vi "Create Event List.vi"(10 "Event Outcome":T1, 11 "Array in":T1[](array[typedef])) -> (3 "Array out":T1[](array[typedef]))   [LabVIEW 2017]
uses:
  state-manager/Event.ctl
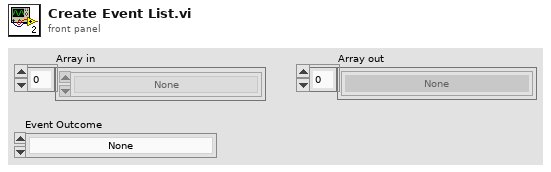
[diagram p1: front panel]
types:
  T1 = typedef "Event.ctl" = enum16{"None", "Zig Zag Finished", "Start Obstacle Avoidance", "Start Button Pressed", "Black & Yellow Tape Touched", "Black & Yellow Tape Passed", "Green Tape Crossed", "Red Tape Touched", "Rough Terrain Touched", "Black Tape Crossed", "Tape Edge Too Close", "Wall Too Close", "Rough Terrain Passed", "Ramp Passed", "Stop Button Pressed", "Recentered", "End Zone Wait Timed Out"}
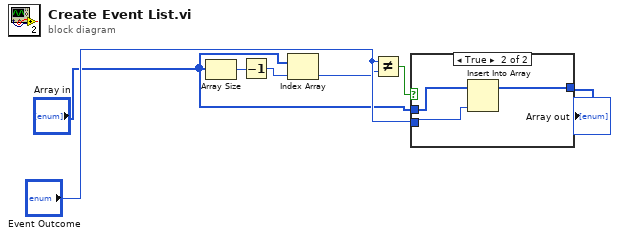
[diagram p0: block diagram]
diagram:
  n1 = Array Size(array="Array in") -> (size(s)=w1:i32)
  n2 = Decrement(x=w1) -> (x-1=w2:i32)
  n3 = Index Array(array="Array in", index=w2) -> (element=w3:T1)
  n4 = Not Equal?(x="Event Outcome", y=w3) -> (x != y?=w4:bool)
  n5 = case shown="True" w4 {
    tunnel: "Array in" -> [w8 w11]
    tunnel: "Event Outcome" -> [_ w10]
    tunnel: [w8 w9] -> w7
    frame False {
    }
    frame True {
      n6 = Insert Into Array(array=w11, new element=w10) -> (w9:T1[])  [unwired: 1 in]
    }
  }
  "Array out" <- w7
